vi "FPGA_MAIN.vi"() -> ()   [LabVIEW 2009]
doc: "IRQ Guide:\n3 - SICK IRQ - used to wait at the beginning to set baud rate, and then later to ask for data from the SICK.\n4 - Simple Serial Read IRQ - Used to wait at the beginning to set GPS port baud rate, and then later used to read a data byte from the serial port.\n5 - Simple Serial Clear RX FIFO IRQ - Used to clear the GPS port rx FIFO"
uses:
  <vilib>/LabVIEW Targets/FPGA/cRIO/shared/nicrio_ModuleControls/nicrio_cRIO-9871_BaudRateEnum.ctl
  <vilib>/LabVIEW Targets/FPGA/cRIO/shared/nicrio_ModuleControls/nicrio_cRIO-9871_DataBitsEnum.ctl
  <vilib>/LabVIEW Targets/FPGA/cRIO/shared/nicrio_ModuleControls/nicrio_cRIO-9871_StopBitsEnum.ctl
  <vilib>/LabVIEW Targets/FPGA/cRIO/shared/nicrio_ModuleControls/nicrio_cRIO-9871_ParityEnum.ctl
  <vilib>/LabVIEW Targets/FPGA/cRIO/shared/nicrio_ModuleControls/nicrio_cRIO-9871_FlowControlEnum.ctl
  <vilib>/eio/EIONode/EIONode.xnode
  <vilib>/rvi/eio/nirviEIOImplementation/nirviEIOImplementation.xnode
  <vilib>/rvi/eio/common/nirviEmuTemplateMethod_noerrors.vi
  <vilib>/rvi/eio/common/nirviEmuClasses.ctl
  <vilib>/rvi/Arithmetic/AddSubMult/XNode/nirviSatArithmetic.xnode
  <vilib>/rvi/DataTransferAndStorage/Container/XNode/niFpgaContainer.xnode
  <vilib>/rvi/interface/RandomDataEmulation/niFpgaRandomDataHandleErrors.vi
  <vilib>/rvi/interface/RandomDataEmulation/nirviRandomDataFPGAFIFO.vi
  <vilib>/rvi/DataTransferAndStorage/Container/Common/niFpgaContainerMethod.ctl
  <vilib>/rvi/DataTransferAndStorage/Container/Common/niFpgaTransferTypeControl.ctl
  <vilib>/rvi/Memory/Memory_Emulation/nirvimemoryEmulationManagerCache_GetValue.vi
  <vilib>/rvi/Memory/Memory_Emulation/nirvimemoryEmulationManagerCache_InsertValue.vi
  <vilib>/rvi/DataTransferAndStorage/Container/Common/niFpgaContainerGetUniqueNameForEmu.vi
  <vilib>/Utility/error.llb/Clear Errors.vi
  <vilib>/rvi/Memory/Memory_Emulation/nirvimemoryEmulationManagerCache_SetValue.vi
  <vilib>/eio/EIOPropertyNode/EIOPropertyNode.xnode
  <vilib>/rvi/eio/nirviEIOPropertyImplementation/nirviEIOPropertyImplementation.xnode
  <vilib>/rvi/eio/common/nirviEmuTemplatePropertySet_errors.vi
  <vilib>/eio/EIOMethodNode/EIOMethodNode.xnode
  <vilib>/rvi/eio/nirviEIOMethodImplementation/nirviEIOMethodImplementation.xnode
  <vilib>/rvi/eio/common/nirviEmuTemplateMethod_errors.vi
  SICK VI's/SICK Reader States.ctl
  <vilib>/rvi/eio/common/nirviEmuTemplatePropertyGet_errors.vi
panel:
  in  "Position Reset":bool
  in  "Velocity Interval (uSec)":u32=1000
  out "Right Position (Counts)":i32
  out "Right Acceleration (Counts/Interval)":i32
  out "Right Velocity (Counts/Interval)":i32
  out "Left Position (Counts)":i32
  out "Left Acceleration (Counts/Interval)":i32
  out "Left Velocity (Counts/Interval)":i32
  in  "Safety Light LED ON/OFF/BLINK":u8
  in  "That Was Easy Duration":u32 caption="That Was Easy Duration (ms)"
  in  "Mod2/DIO15:8":u8
  out "Waveform Chart (Turn)":i32(graph)
  out "High Pulse Length (Turn)":i32
  out "Low Pulse Length (Turn)":i32
  out "Pulse Period (Turn)":i32
  out "Waveform Chart (Throttle)":i32(graph)
  out "High Pulse Length (Throttle)":i32
  out "Low Pulse Length (Throttle)":i32
  out "Pulse Period (Throttle)":i32
  out "Debounced BTTN1":bool
  out "Debounced SW2":bool
  out "Debounced SW1":bool
  in  "LED7 ON/OFF/BLINK":u8
  in  "LED6 ON/OFF/BLINK":u8
  in  "LED5 ON/OFF/BLINK":u8
  in  "LED4 ON/OFF/BLINK":u8
  in  "LED3 ON/OFF/BLINK":u8
  in  "LED2 ON/OFF/BLINK":u8
  in  "LED1 ON/OFF/BLINK":u8
  in  "GO LED ON/OFF/BLINK":u8
  in  "Safety LED ON/OFF/BLINK":u8
  in  "Sleep":bool
  out "Chassis Temperature":i16
  out "Output Started":bool
  out "Output Halted":bool
  in  "GPS Read Timeout (us)":i32
  out "Bytes at Port?":bool
  out "Current Buffer":u8[](array[numeric])
  out "GPS Data":u8[](array[numeric])
  out "New GPS Data":bool
  out "GPS error out":errorcluster
  out "Analog Readings":fxp<+/-,16,7>[](array[numeric]) format="%.12g"
  out "Debounced Init Switch":bool
  out "Debounced Go Button":bool
  out "Debounced Safety Switch":bool
  in  "Debounce Timeout":i32=100
  in  "LED Multiple":u32=500
  in  "Init LED ON/OFF/BLINK":u8
  in  "EN mask overflow bytes":bool
  in  "En overflow replacement":bool
  out "Read Period":u32
  out "Tick count":u32
  out "error out 2":errorcluster
  out "Read data error":errorcluster
  in  "Read/Write Timeout (ms)":i32
  in  "Bytes at Port Timeout (us)":i32
  in  "Overflow Reading":u16
  out "No Data (timeout)":bool
  out "Correct Response Read?":bool
  out "Current response length":u8
  out "Timed Out":bool
  out "Initialization error":errorcluster
  in  "Set new baud rate wait (usec)":u32
  out "Baud Rate":T1=enum."38.4 kbps"
  out "RT commands timeout":bool
  out "Pre-initialization error":errorcluster
  out "Commands stored":bool
  out "Pre-initialization success":bool
  out "Initialization success":bool
  out "Compass Period (ms)":u16
  in  "Compass Tick Count(mSec)":u16
  out "Compass Heartbeat":bool
  out "Compass comma count":i32
  out "Compass read count":i32
  in  "Compass Timeout (ms)":i32=150
  out "Compass error out":errorcluster
  out "pitch buffer":u8[](array[numeric])
  out "heading data":u8[](array[numeric])
  out "heading buffer":u8[](array[numeric])
  out "roll data":u8[](array[numeric])
  out "roll buffer":u8[](array[numeric])
  out "pitch data":u8[](array[numeric])
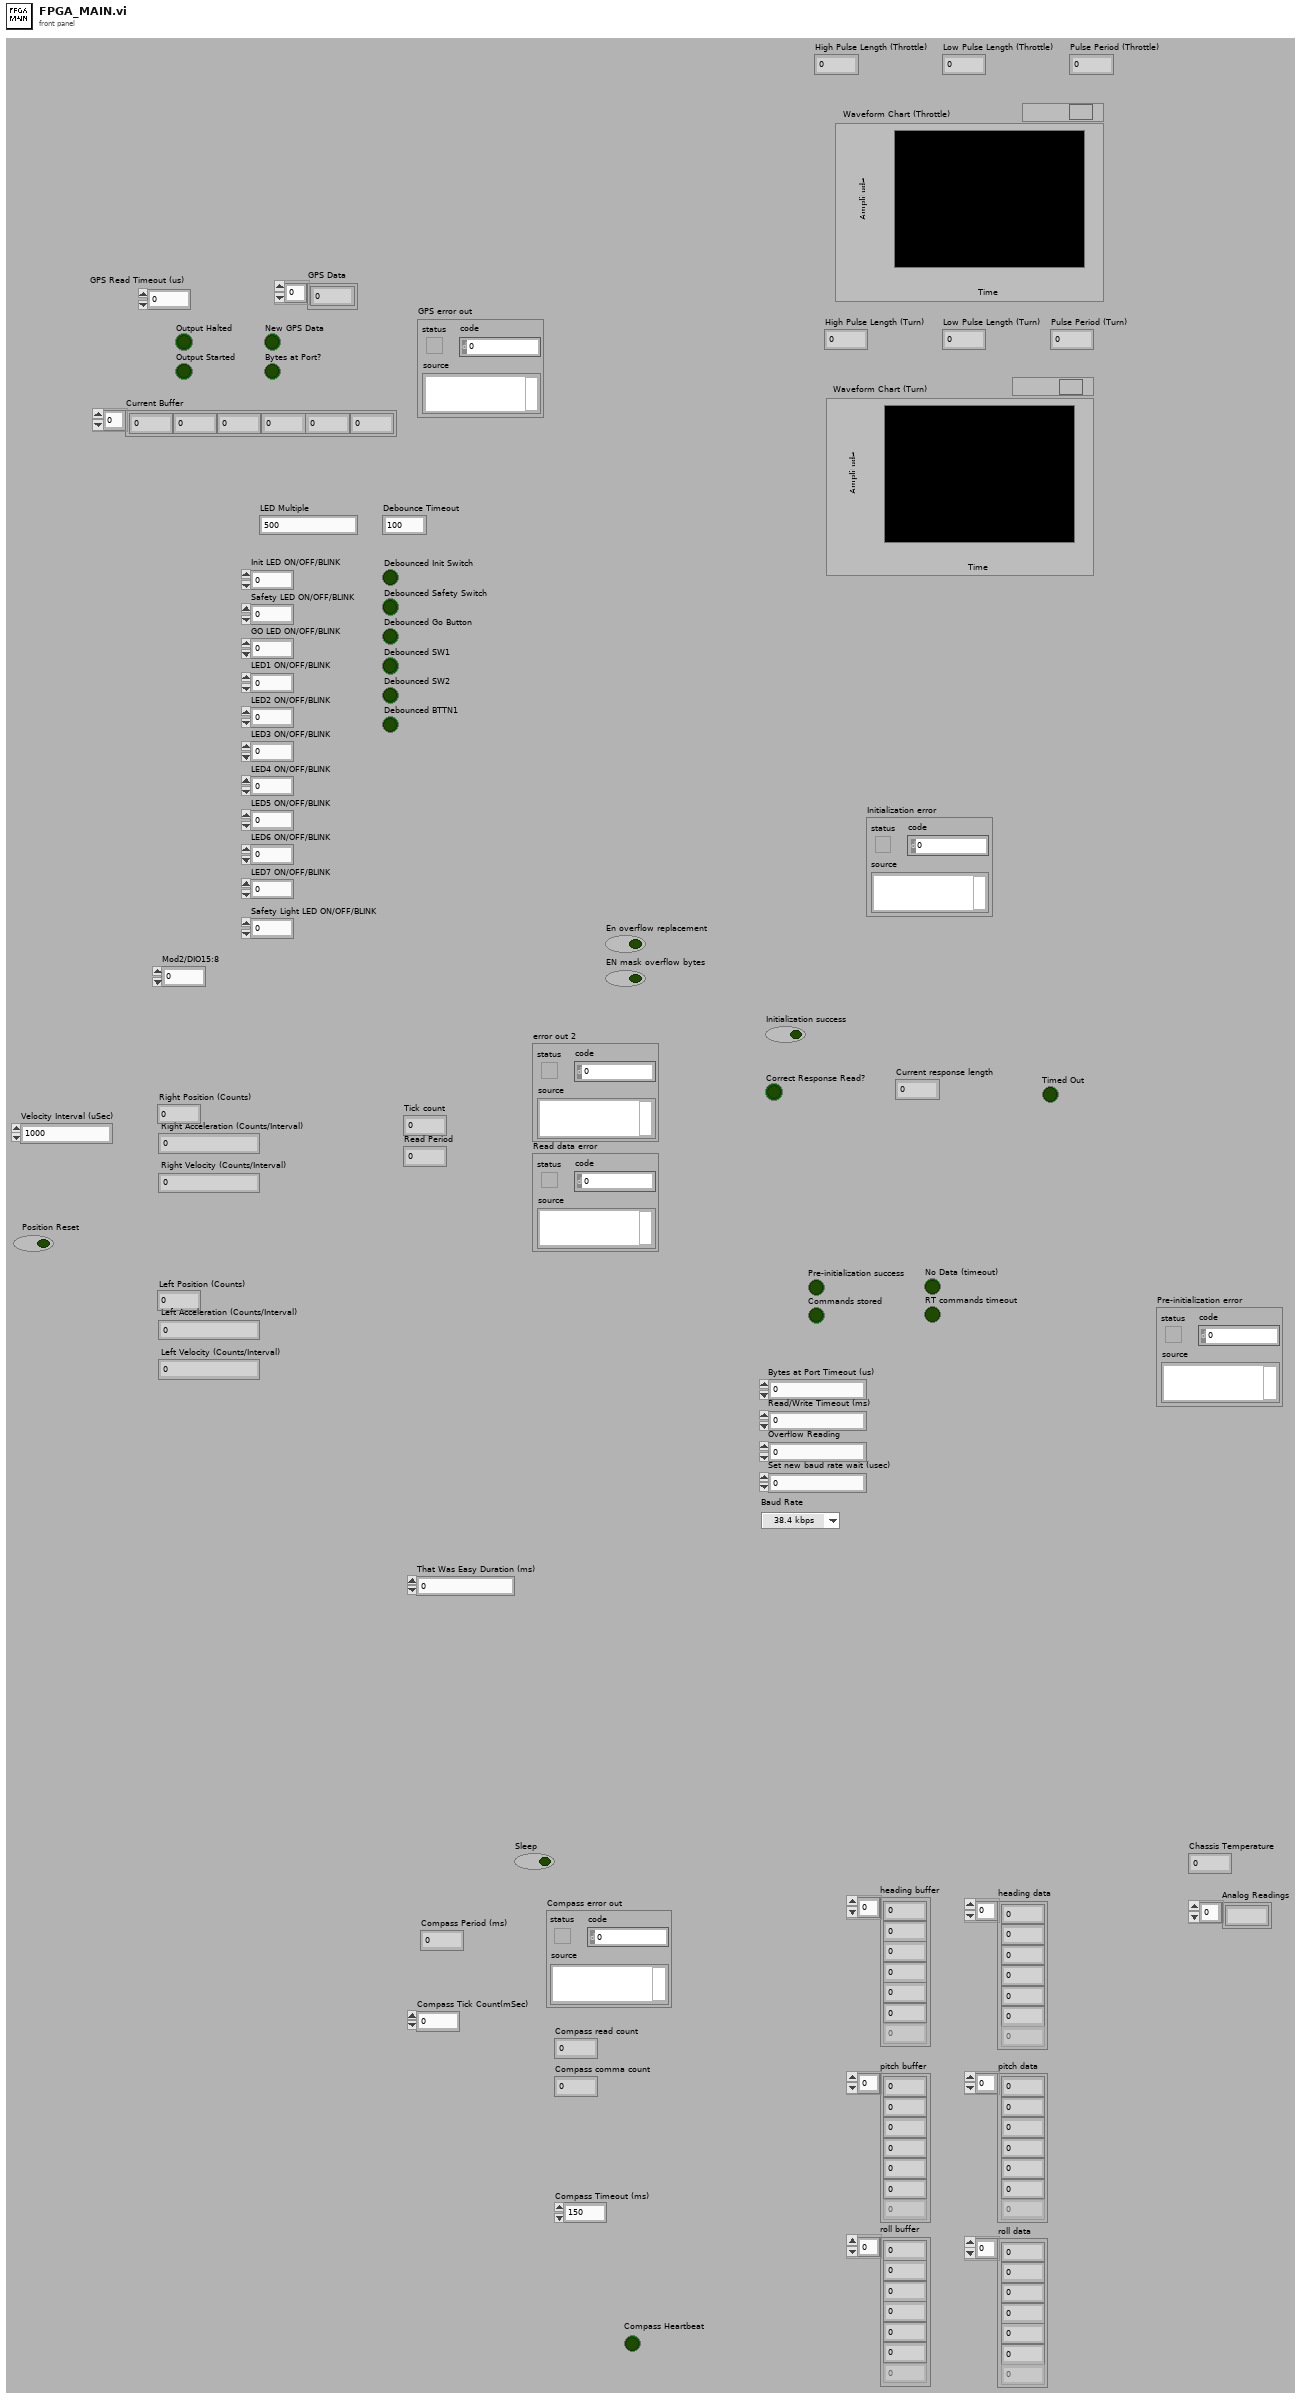
[diagram p1: front panel]
types:
  T1 = typedef "nicrio_cRIO-9871_BaudRateEnum.ctl" = enum16{"75 bps", "110 bps", "134 bps", "150 bps", "300 bps", "600 bps", "1200 bps", "1800 bps", "2400 bps", "4800 bps", "7200 bps", "9600 bps", "14.4 kbps", "19.2 kbps", "28.8 kbps", "38.4 kbps", "57.6 kbps", "115.2 kbps", "230.4 kbps", "460.8 kbps", "921.6 kbps"}
  T2 = typedef "nicrio_cRIO-9871_FlowControlEnum.ctl" = enum8{"None", "Software (XON / XOFF)", "Hardware (RTS / CTS)"}
  T3 = typedef "nicrio_cRIO-9871_ParityEnum.ctl" = enum8{"None", "Odd", "Even", "Mark", "Space"}
  T4 = typedef "nicrio_cRIO-9871_StopBitsEnum.ctl" = enum8{"1", "1.5", "2"}
  T5 = typedef "nicrio_cRIO-9871_DataBitsEnum.ctl" = enum8{"5", "6", "7", "8"}
  T6 = typedef "nirviEmuClasses.ctl" = enum16{"IO Read", "IO Write", "Method", "Property Read", "Property Write"}
  T7 = typedef "niFpgaContainerMethod.ctl" = enum16{"Write", "Read", "Clear", "Get Number of Elements to Write", "Get Number of Elements to Read", "Enable", "Disable", "Flush and Disable", "Get Stream State"}
  T8 = typedef "niFpgaTransferTypeControl.ctl" = enum16{"Target-Scoped", "Host to Target - DMA", "Target to Host - DMA", "Peer to Peer Reader", "Peer to Peer Writer", "Bidirectional"}
  T9 = typedef "SICK Reader States.ctl" = enum16{"Search for 02", "Search for Header", "Read Data"}
  T10 = enum16{"Search for LF", "Read heading", "Read pitch", "Read roll"}
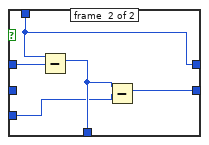
[diagram p2: hidden frame]
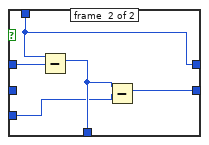
[diagram p3: hidden frame]
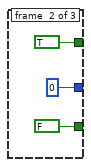
[diagram p4: hidden frame]
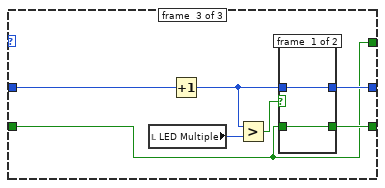
[diagram p5: hidden frame]
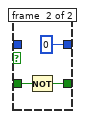
[diagram p6: hidden frame]
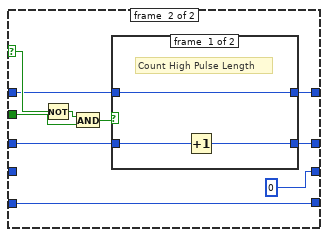
[diagram p8: hidden frame]
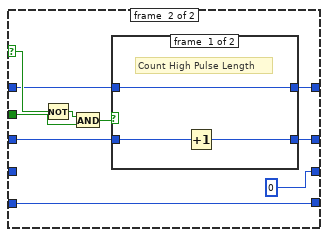
[diagram p11: hidden frame]
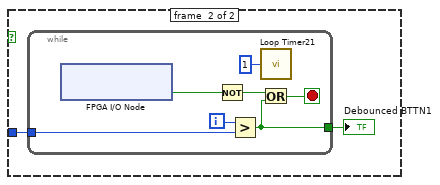
[diagram p13: hidden frame]
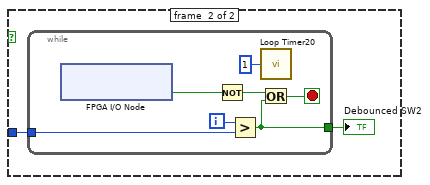
[diagram p14: hidden frame]
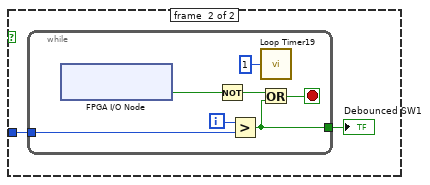
[diagram p15: hidden frame]
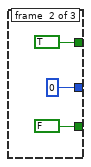
[diagram p16: hidden frame]
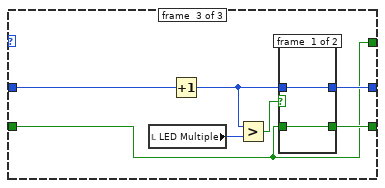
[diagram p17: hidden frame]
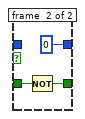
[diagram p18: hidden frame]
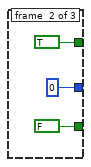
[diagram p19: hidden frame]
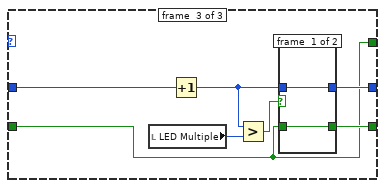
[diagram p20: hidden frame]
diagram:
  # "Debouncing Loops"
  n1 = while "LED3 Loop" {
    shift-right: [w52] -> _
    shift-left: u32 0 -> [w53]
    shift-right: [w51] -> _
    shift-left: FALSE -> [w50]
    stop <- FALSE stop-if-true
    n2 = call "Loop Timer14"("Count(mSec)"=u8 1 ("LED Control Loop Period")) -> ()  [unwired: 1 out]
    n3 = case shown="2" "LED3 ON/OFF/BLINK" {
      tunnel: w53 -> [_ _ w77]
      tunnel: [u32 0 u32 0 w76] -> w52
      tunnel: [FALSE FALSE w73] -> w51
      tunnel: w50 -> [_ _ w72]
      tunnel: [FALSE TRUE w72] -> w49
      frame #0 {
      }
      frame #1 {
      }
      frame #2 {
        n4 = local read "LED Multiple"() -> (w71:u32)
        n5 = Increment(x=w77) -> (x+1=w75:u32)
        n6 = Greater?(x=w75, y=w71) -> (0:w74:bool)
        n7 = case shown="True" w74 {
          tunnel: [w79 u32 0] -> w76
          tunnel: w75 -> [w79 _]
          tunnel: [w78 w81] -> w73
          tunnel: w72 -> [w78 w80]
          frame #0 {
          }
          frame #1 {
            n8 = Not(x=w80) -> (.not. x?=w81:bool)
          }
        }
      }
    }
    n9 = xnode "FPGA I/O Node"("Mod2/DIO24"=w49) -> ()  [unwired: 1 in, 1 out]
  }
  n10 = while "LED4 Loop" {
    shift-right: [w89] -> _
    shift-left: u32 0 -> [w90]
    shift-right: [w88] -> _
    shift-left: FALSE -> [w87]
    stop <- FALSE stop-if-true
    n11 = call "Loop Timer15"("Count(mSec)"=u8 1 ("LED Control Loop Period")) -> ()  [unwired: 1 out]
    n12 = case shown="2" "LED4 ON/OFF/BLINK" {
      tunnel: w90 -> [_ _ w114]
      tunnel: [u32 0 u32 0 w113] -> w89
      tunnel: [FALSE FALSE w110] -> w88
      tunnel: w87 -> [_ _ w109]
      tunnel: [FALSE TRUE w109] -> w86
      frame #0 {
      }
      frame #1 {
      }
      frame #2 {
        n13 = local read "LED Multiple"() -> (w108:u32)
        n14 = Increment(x=w114) -> (x+1=w112:u32)
        n15 = Greater?(x=w112, y=w108) -> (0:w111:bool)
        n16 = case shown="True" w111 {
          tunnel: [w116 u32 0] -> w113
          tunnel: w112 -> [w116 _]
          tunnel: [w115 w118] -> w110
          tunnel: w109 -> [w115 w117]
          frame #0 {
          }
          frame #1 {
            n17 = Not(x=w117) -> (.not. x?=w118:bool)
          }
        }
      }
    }
    n18 = xnode "FPGA I/O Node"("Mod2/DIO25"=w86) -> ()  [unwired: 1 in, 1 out]
  }
  n19 = while "LED5 Loop" {
    shift-right: [w126] -> _
    shift-left: u32 0 -> [w127]
    shift-right: [w125] -> _
    shift-left: FALSE -> [w124]
    stop <- FALSE stop-if-true
    n20 = call "Loop Timer16"("Count(mSec)"=u8 1 ("LED Control Loop Period")) -> ()  [unwired: 1 out]
    n21 = case shown="2" "LED5 ON/OFF/BLINK" {
      tunnel: w127 -> [_ _ w151]
      tunnel: [u32 0 u32 0 w150] -> w126
      tunnel: [FALSE FALSE w147] -> w125
      tunnel: w124 -> [_ _ w146]
      tunnel: [FALSE TRUE w146] -> w123
      frame #0 {
      }
      frame #1 {
      }
      frame #2 {
        n22 = local read "LED Multiple"() -> (w145:u32)
        n23 = Increment(x=w151) -> (x+1=w149:u32)
        n24 = Greater?(x=w149, y=w145) -> (0:w148:bool)
        n25 = case shown="True" w148 {
          tunnel: [w153 u32 0] -> w150
          tunnel: w149 -> [w153 _]
          tunnel: [w152 w155] -> w147
          tunnel: w146 -> [w152 w154]
          frame #0 {
          }
          frame #1 {
            n26 = Not(x=w154) -> (.not. x?=w155:bool)
          }
        }
      }
    }
    n27 = xnode "FPGA I/O Node"("Mod2/DIO26"=w123) -> ()  [unwired: 1 in, 1 out]
  }
  n28 = while "LED6 Loop" {
    shift-right: [w163] -> _
    shift-left: u32 0 -> [w164]
    shift-right: [w162] -> _
    shift-left: FALSE -> [w161]
    stop <- FALSE stop-if-true
    n29 = call "Loop Timer17"("Count(mSec)"=u8 1 ("LED Control Loop Period")) -> ()  [unwired: 1 out]
    n30 = case shown="2" "LED6 ON/OFF/BLINK" {
      tunnel: w164 -> [_ _ w188]
      tunnel: [u32 0 u32 0 w187] -> w163
      tunnel: [FALSE FALSE w184] -> w162
      tunnel: w161 -> [_ _ w183]
      tunnel: [FALSE TRUE w183] -> w160
      frame #0 {
      }
      frame #1 {
      }
      frame #2 {
        n31 = local read "LED Multiple"() -> (w182:u32)
        n32 = Increment(x=w188) -> (x+1=w186:u32)
        n33 = Greater?(x=w186, y=w182) -> (0:w185:bool)
        n34 = case shown="True" w185 {
          tunnel: [w190 u32 0] -> w187
          tunnel: w186 -> [w190 _]
          tunnel: [w189 w192] -> w184
          tunnel: w183 -> [w189 w191]
          frame #0 {
          }
          frame #1 {
            n35 = Not(x=w191) -> (.not. x?=w192:bool)
          }
        }
      }
    }
    n36 = xnode "FPGA I/O Node"("Mod2/DIO29"=w160) -> ()  [unwired: 1 in, 1 out]
  }
  n37 = while "LED7 Loop" {
    shift-right: [w200] -> _
    shift-left: u32 0 -> [w201]
    shift-right: [w199] -> _
    shift-left: FALSE -> [w198]
    stop <- FALSE stop-if-true
    n38 = call "Loop Timer18"("Count(mSec)"=u8 1 ("LED Control Loop Period")) -> ()  [unwired: 1 out]
    n39 = case shown="2" "LED7 ON/OFF/BLINK" {
      tunnel: w201 -> [_ _ w225]
      tunnel: [u32 0 u32 0 w224] -> w200
      tunnel: [FALSE FALSE w221] -> w199
      tunnel: w198 -> [_ _ w220]
      tunnel: [FALSE TRUE w220] -> w197
      frame #0 {
      }
      frame #1 {
      }
      frame #2 {
        n40 = local read "LED Multiple"() -> (w219:u32)
        n41 = Increment(x=w225) -> (x+1=w223:u32)
        n42 = Greater?(x=w223, y=w219) -> (0:w222:bool)
        n43 = case shown="True" w222 {
          tunnel: [w227 u32 0] -> w224
          tunnel: w223 -> [w227 _]
          tunnel: [w226 w229] -> w221
          tunnel: w220 -> [w226 w228]
          frame #0 {
          }
          frame #1 {
            n44 = Not(x=w228) -> (.not. x?=w229:bool)
          }
        }
      }
    }
    n45 = xnode "FPGA I/O Node"("Mod2/DIO30"=w197) -> ()  [unwired: 1 in, 1 out]
  }
  n46 = while {
    stop <- FALSE stop-if-true
    n47 = xnode "FPGA I/O Node"() -> ("Mod1/AI0"=w245:fxp<+/-,16,7>)  [unwired: 1 in, 1 out]
    n48 = xnode "FPGA I/O Node"() -> ("Mod1/AI1"=w244:fxp<+/-,16,7>)  [unwired: 1 in, 1 out]
    n49 = xnode "FPGA I/O Node"() -> ("Mod1/AI2"=w243:fxp<+/-,16,7>)  [unwired: 1 in, 1 out]
    n50 = xnode "FPGA I/O Node"() -> ("Mod1/AI3"=w242:fxp<+/-,16,7>)  [unwired: 1 in, 1 out]
    n51 = xnode "FPGA I/O Node"() -> ("Mod1/AI4"=w241:fxp<+/-,16,7>)  [unwired: 1 in, 1 out]
    n52 = xnode "FPGA I/O Node"() -> ("Mod1/AI5"=w240:fxp<+/-,16,7>)  [unwired: 1 in, 1 out]
    n53 = xnode "FPGA I/O Node"() -> ("Mod1/AI6"=w239:fxp<+/-,16,7>)  [unwired: 1 in, 1 out]
    n54 = xnode "FPGA I/O Node"() -> ("Mod1/AI7"=w238:fxp<+/-,16,7>)  [unwired: 1 in, 1 out]
    n55 = xnode "FPGA I/O Node"() -> ("Chassis Temperature"=→"Chassis Temperature":i16)  [unwired: 1 in, 1 out]
    n56 = xnode "FPGA I/O Node"("Sleep"="Sleep") -> ()  [unwired: 1 in, 1 out]
    n57 = Build Array(w245, w244, w243, w242, w241, w240, w239, w238) -> (→"Analog Readings":fxp<+/-,16,7>[])
    n58 = Number To Boolean Array(number="Mod2/DIO15:8") -> (Boolean array=w235:bool[])
    n59 = Index Array(array=w235, index #1=1 ("index")) -> (element #1=w232:bool, element #2=w231:bool)  [unwired: 1 in]
    n60 = xnode "FPGA I/O Node"("Mod2/DIO13"=w232, "Mod2/DIO14"=w231) -> ()  [unwired: 2 in, 2 out]
  }
  n61 = while "LED2 Loop" {
    shift-right: [w466] -> _
    shift-left: u32 0 -> [w467]
    shift-right: [w465] -> _
    shift-left: FALSE -> [w464]
    stop <- FALSE stop-if-true
    n62 = call "Loop Timer13"("Count(mSec)"=u8 1 ("LED Control Loop Period")) -> ()  [unwired: 1 out]
    n63 = case shown="2" "LED2 ON/OFF/BLINK" {
      tunnel: w467 -> [_ _ w491]
      tunnel: [u32 0 u32 0 w490] -> w466
      tunnel: [FALSE FALSE w487] -> w465
      tunnel: w464 -> [_ _ w486]
      tunnel: [FALSE TRUE w486] -> w463
      frame #0 {
      }
      frame #1 {
      }
      frame #2 {
        n64 = local read "LED Multiple"() -> (w485:u32)
        n65 = Increment(x=w491) -> (x+1=w489:u32)
        n66 = Greater?(x=w489, y=w485) -> (0:w488:bool)
        n67 = case shown="True" w488 {
          tunnel: [w493 u32 0] -> w490
          tunnel: w489 -> [w493 _]
          tunnel: [w492 w495] -> w487
          tunnel: w486 -> [w492 w494]
          frame #0 {
          }
          frame #1 {
            n68 = Not(x=w494) -> (.not. x?=w495:bool)
          }
        }
      }
    }
    n69 = xnode "FPGA I/O Node"("Mod2/DIO23"=w463) -> ()  [unwired: 1 in, 1 out]
  }
  n70 = while "Safety Light LED Loop" {
    shift-right: [w503] -> _
    shift-left: u32 0 -> [w504]
    shift-right: [w502] -> _
    shift-left: FALSE -> [w501]
    stop <- FALSE stop-if-true
    n71 = call "Loop Timer24"("Count(mSec)"=u8 1 ("LED Control Loop Period")) -> ()  [unwired: 1 out]
    n72 = case shown="0" "Safety Light LED ON/OFF/BLINK" {
      tunnel: w504 -> [_ _ w528]
      tunnel: [u32 0 u32 0 w527] -> w503
      tunnel: [FALSE FALSE w524] -> w502
      tunnel: w501 -> [_ _ w523]
      tunnel: [FALSE TRUE w523] -> w500
      frame #0 {
      }
      frame #1 {
      }
      frame #2 {
        n73 = local read "LED Multiple"() -> (w522:u32)
        n74 = Increment(x=w528) -> (x+1=w526:u32)
        n75 = Greater?(x=w526, y=w522) -> (0:w525:bool)
        n76 = case shown="True" w525 {
          tunnel: [w530 u32 0] -> w527
          tunnel: w526 -> [w530 _]
          tunnel: [w529 w532] -> w524
          tunnel: w523 -> [w529 w531]
          frame #0 {
          }
          frame #1 {
            n77 = Not(x=w531) -> (.not. x?=w532:bool)
          }
        }
      }
    }
    n78 = xnode "FPGA I/O Node"("Mod2/DIO15"=w500) -> ()  [unwired: 1 in, 1 out]
  }
  n79 = while "GO LED Loop" {
    shift-right: [w540] -> _
    shift-left: u32 0 -> [w541]
    shift-right: [w539] -> _
    shift-left: FALSE -> [w538]
    stop <- FALSE stop-if-true
    # "GO LED"
    n80 = call "Loop Timer11"("Count(mSec)"=u8 1 ("LED Control Loop Period")) -> ()  [unwired: 1 out]
    n81 = case shown="0, Default" "GO LED ON/OFF/BLINK" {
      tunnel: w541 -> [_ _ w565]
      tunnel: [u32 0 u32 0 w564] -> w540
      tunnel: [FALSE FALSE w561] -> w539
      tunnel: w538 -> [_ _ w560]
      tunnel: [FALSE TRUE w560] -> w537
      frame #0 {
      }
      frame #1 {
      }
      frame #2 {
        n82 = local read "LED Multiple"() -> (w559:u32)
        n83 = Increment(x=w565) -> (x+1=w563:u32)
        n84 = Greater?(x=w563, y=w559) -> (0:w562:bool)
        n85 = case shown="True" w562 {
          tunnel: [w567 u32 0] -> w564
          tunnel: w563 -> [w567 _]
          tunnel: [w566 w569] -> w561
          tunnel: w560 -> [w566 w568]
          frame #0 {
          }
          frame #1 {
            n86 = Not(x=w568) -> (.not. x?=w569:bool)
          }
        }
      }
    }
    n87 = xnode "FPGA I/O Node"("Mod2/DIO18"=w537) -> ()  [unwired: 1 in, 1 out]
  }
  n88 = while "LED1 Loop" {
    shift-right: [w577] -> _
    shift-left: u32 0 -> [w578]
    shift-right: [w576] -> _
    shift-left: FALSE -> [w575]
    stop <- FALSE stop-if-true
    n89 = call "Loop Timer12"("Count(mSec)"=u8 1 ("LED Control Loop Period")) -> ()  [unwired: 1 out]
    n90 = case shown="2" "LED1 ON/OFF/BLINK" {
      tunnel: w578 -> [_ _ w602]
      tunnel: [u32 0 u32 0 w601] -> w577
      tunnel: [FALSE FALSE w598] -> w576
      tunnel: w575 -> [_ _ w597]
      tunnel: [FALSE TRUE w597] -> w574
      frame #0 {
      }
      frame #1 {
      }
      frame #2 {
        n91 = local read "LED Multiple"() -> (w596:u32)
        n92 = Increment(x=w602) -> (x+1=w600:u32)
        n93 = Greater?(x=w600, y=w596) -> (0:w599:bool)
        n94 = case shown="True" w599 {
          tunnel: [w604 u32 0] -> w601
          tunnel: w600 -> [w604 _]
          tunnel: [w603 w606] -> w598
          tunnel: w597 -> [w603 w605]
          frame #0 {
          }
          frame #1 {
            n95 = Not(x=w605) -> (.not. x?=w606:bool)
          }
        }
      }
    }
    n96 = xnode "FPGA I/O Node"("Mod2/DIO22"=w574) -> ()  [unwired: 1 in, 1 out]
  }
  n97 = while "Safety LED Loop" {
    shift-right: [w614] -> _
    shift-left: u32 0 -> [w615]
    shift-right: [w613] -> _
    shift-left: FALSE -> [w612]
    stop <- FALSE stop-if-true
    # "Safety LED"
    n98 = call "Loop Timer10"("Count(mSec)"=u8 1 ("LED Control Loop Period")) -> ()  [unwired: 1 out]
    n99 = case shown="2" "Safety LED ON/OFF/BLINK" {
      tunnel: w615 -> [_ _ w639]
      tunnel: [u32 0 u32 0 w638] -> w614
      tunnel: [FALSE FALSE w635] -> w613
      tunnel: w612 -> [_ _ w634]
      tunnel: [FALSE TRUE w634] -> w611
      frame #0 {
      }
      frame #1 {
      }
      frame #2 {
        n100 = local read "LED Multiple"() -> (w633:u32)
        n101 = Increment(x=w639) -> (x+1=w637:u32)
        n102 = Greater?(x=w637, y=w633) -> (0:w636:bool)
        n103 = case shown="True" w636 {
          tunnel: [w641 u32 0] -> w638
          tunnel: w637 -> [w641 _]
          tunnel: [w640 w643] -> w635
          tunnel: w634 -> [w640 w642]
          frame #0 {
          }
          frame #1 {
            n104 = Not(x=w642) -> (.not. x?=w643:bool)
          }
        }
      }
    }
    n105 = xnode "FPGA I/O Node"("Mod2/DIO17"=w611) -> ()  [unwired: 1 in, 1 out]
  }
  n106 = while "Init LED Loop" {
    shift-right: [w651] -> _
    shift-left: u32 0 -> [w652]
    shift-right: [w650] -> _
    shift-left: FALSE -> [w649]
    stop <- FALSE stop-if-true
    # "Init LED"
    n107 = call "Loop Timer4"("Count(mSec)"=u8 1 ("LED Control Loop Period")) -> ()  [unwired: 1 out]
    n108 = case shown="2" "Init LED ON/OFF/BLINK" {
      tunnel: w652 -> [_ _ w676]
      tunnel: [u32 0 u32 0 w675] -> w651
      tunnel: [FALSE FALSE w672] -> w650
      tunnel: w649 -> [_ _ w671]
      tunnel: [FALSE TRUE w671] -> w648
      frame #0 {
      }
      frame #1 {
      }
      frame #2 {
        n109 = local read "LED Multiple"() -> (w670:u32)
        n110 = Increment(x=w676) -> (x+1=w674:u32)
        n111 = Greater?(x=w674, y=w670) -> (0:w673:bool)
        n112 = case shown="True" w673 {
          tunnel: [w678 u32 0] -> w675
          tunnel: w674 -> [w678 _]
          tunnel: [w677 w680] -> w672
          tunnel: w671 -> [w677 w679]
          frame #0 {
          }
          frame #1 {
            n113 = Not(x=w679) -> (.not. x?=w680:bool)
          }
        }
      }
    }
    n114 = xnode "FPGA I/O Node"("Mod2/DIO16"=w648) -> ()  [unwired: 1 in, 1 out]
  }
  n115 = while {
    stop <- FALSE stop-if-true
    n116 = flat-sequence {
      tunnel: [w688] -> w685
      tunnel: w685 -> [w928]
      tunnel: [w927] -> w683
      tunnel: w683 -> [w945]
      tunnel: [w945] -> w682
      tunnel: w682 -> [w1198]
      frame #0 {
        w686 = FALSE ("Initialization complete")
        n117 = local write "RT commands timeout"(w686) -> ()
        n118 = local write "Pre-initialization success"(w686) -> ()
        n119 = local write "Commands stored"(w686) -> ()
        n120 = local write "No Data (timeout)"(w686) -> ()
        "Initialization success" <- w686
      }
      frame #1 {
        n121 = flat-sequence {
          tunnel: [w863] -> w687
          tunnel: [TRUE] -> w689
          frame #0 {
            w865 = nicrio_cRIO-9871_BaudRateEnum."38.4 kbps" ("Baud Rate")
            # "Set baud rate to 38.4 kbps and tell it to cease continuous data output to prevent the FPGA from mixing up data messages and command responses"
            n122 = call "Wait"("Count(uSec)"="Set new baud rate wait (usec)") -> ()  [unwired: 1 out]
            n123 = xnode "FPGA I/O Property Node"("Baud Rate"=w865, "Data Bits"=nicrio_cRIO-9871_DataBitsEnum."8", "Stop Bits"=nicrio_cRIO-9871_StopBitsEnum."1", "Parity"=nicrio_cRIO-9871_ParityEnum."None", "Flow Control"=nicrio_cRIO-9871_FlowControlEnum."None") -> ("error out"=w862:errorcluster)  [unwired: 2 in, 1 out]
            n124 = xnode "FPGA I/O Method Node"("error in"=w862) -> ("error out"=w863:errorcluster)  [unwired: 1 in, 1 out]
            "Baud Rate" <- w865
          }
        }
        n125 = flat-sequence {
          tunnel: errorcluster {"status"=FALSE, "code"=0, "source"=""} ("error out") -> [w694]
          tunnel: [w694] -> w693
          tunnel: w693 -> [w699]
          tunnel: [w698] -> w691
          tunnel: [TRUE] -> w690
          frame #0 {
            n126 = call "Interrupt"("Wait Until Cleared"=TRUE, "IRQ Number"=u8 3) -> ()  [unwired: 1 out]
          }
          frame #1 {
            n127 = for "Read all the commands from the RT to memory" {
              N: 160 -> [_]
              tunnel: w699 -> [w706]
              tunnel: [w705] -> w698
              i -> [w702]
              n128 = local read "Read/Write Timeout (ms)"() -> (w704:i32)
              n129 = xnode ("FIFO Read")("Timeout"=w704, "error in (no error)"=w706) -> ("Element"=w708:u8, "Timed Out?"=→"RT commands timeout":bool, "error out"=w707:errorcluster)  [unwired: 1 in, 1 out]
              n130 = To Unsigned Long Integer(number=w702) -> (unsigned 32bit integer=w701:u32)
              n131 = xnode ("Memory Write")("Address"=w701, "Data"=w708, "error in (no error)"=w707) -> ("error out"=w705:errorcluster)  [unwired: 1 in, 1 out]
            }
          }
        }
        n132 = Select(t=w687, s=w687, f=w691) -> (s? t:f=w688:errorcluster)
        "Pre-initialization error" <- w688
        "Commands stored" <- w690
        "Pre-initialization success" <- w689
      }
      frame #2 {
        n133 = case shown="No Error" w928 {
          selector: w928 -> [w929 w944]
          tunnel: [w930 w944] -> w927
          frame #0 {
            n134 = for {
              N: 5 -> [_]
              shift-right: [w934] -> w930
              shift-left: w929 -> [w935]
              i -> [w933]
              n135 = To Unsigned Long Integer(number=w933) -> (unsigned 32bit integer=w932:u32)
              n136 = while {
                tunnel: w935 -> [w939]
                tunnel: [w941] -> w934
                tunnel: w932 -> [w936]
                stop <- w942 stop-if-true
                n137 = local read "Read/Write Timeout (ms)"() -> (w937:i32)
                n138 = call "FPGA_SICK Write Command.vi"("error in (no error)"=w939, "Read/Write Timeout (ms)"=w937, "Command index"=w936) -> ("error out"=w938:errorcluster)  [unwired: 8 out]
                n139 = call "FPGA_SICK Read Response.vi"("error in (no error)"=w938, "Timeout (ms)"=w937, "Response Index"=w936) -> ("error out"=w941:errorcluster, "Timed Out"=→"Timed Out":bool, "Current response length"=→"Current response length":u8, "Correct Response Read?"=w942:bool)  [unwired: 5 out]
                "Correct Response Read?" <- w942
              }
            }
          }
          frame #1 {
          }
        }
        "Initialization error" <- w927
      }
      frame #3 {
        n140 = local write "Initialization success"(TRUE ("Initialization complete")) -> ()
        n141 = call "Wait2"("Count(mSec)"=u8 100 ("Count(Ticks)")) -> ()  [unwired: 1 out]
        n142 = for {
          N: 181 -> [_]
          tunnel: u16 0 ("Data") -> [w1073]
          i -> [w1075]
          n143 = To Unsigned Long Integer(number=w1075) -> (unsigned 32bit integer=w1074:u32)
          n144 = xnode ("Memory Write")("Address"=w1074, "Data"=w1073) -> ()  [unwired: 1 in, 1 out]
        }
        n145 = xnode ("Memory Write")("Address"=u32 0, "Data"="Overflow Reading") -> ()  [unwired: 1 in, 1 out]
      }
      frame #4 {
        n146 = case shown="No Error" w1198 {
          selector: w1198 -> [_ w1837]
          tunnel: [w1199 w1837] -> w1197
          frame #0 {
            n147 = while {
              tunnel: errorcluster {"status"=FALSE, "code"=0, "source"=""} ("error out") -> [w1206]
              stop <- FALSE stop-if-true
              n148 = flat-sequence {
                tunnel: w1206 -> [w1208]
                tunnel: [w1208] -> w1207
                tunnel: w1207 -> [w1212]
                tunnel: [w1211] -> w1205
                frame #0 {
                  n149 = call "Interrupt2"("Wait Until Cleared"=TRUE, "IRQ Number"=u8 3) -> ()  [unwired: 1 out]
                }
                frame #1 {
                  n150 = for {
                    N: 181 -> [_]
                    tunnel: w1212 -> [w1218]
                    tunnel: [w1214] -> w1211
                    i -> [w1220]
                    n151 = To Unsigned Long Integer(number=w1220) -> (unsigned 32bit integer=w1219:u32)
                    n152 = xnode ("Memory Read")("Address"=w1219, "error in (no error)"=w1218) -> ("Data"=w1217:u16, "error out"=w1215:errorcluster)  [unwired: 1 in, 1 out]
                    n153 = local read "Read/Write Timeout (ms)"() -> (w1216:i32)
                    n154 = xnode ("FIFO Write")("Element"=w1217, "Timeout"=w1216, "error in (no error)"=w1215) -> ("error out"=w1214:errorcluster)  [unwired: 1 in, 2 out]
                  }
                }
              }
              "error out 2" <- w1205
            }
            n155 = while {
              tunnel: u8[] [128, 110, 1, 176, 181, 0] -> [w1378]
              tunnel: errorcluster {"status"=FALSE, "code"=0, "source"=""} ("error out") -> [w1377]
              shift-right: [w1376] -> _
              shift-left: SICK_Reader_States."Search for 02" ("SICK Reader States") -> [w1379]
              tunnel: [w1375] -> w1199
              stop <- FALSE stop-if-true
              n156 = case shown="\"Read Data\"" w1379 {
                tunnel: w1378 -> [_ w1459 _]
                tunnel: w1377 -> [w1389 w1458 w1546]
                tunnel: [w1387 w1457 w1543] -> w1375
                tunnel: [w1380 w1455 SICK_Reader_States."Search for 02" ("SICK Reader States")] -> w1376
                frame #0 {
                  n157 = while {
                    tunnel: [w1393] -> w1388
                    tunnel: w1389 -> [w1391]
                    i -> [w1395]
                    stop <- w1397 stop-if-true
                    n158 = xnode "FPGA I/O Property Node"("error in"=w1391) -> ("error out"=w1393:errorcluster, "Bytes at Port"=w1398:u8)  [unwired: 1 in, 1 out]
                    n159 = Not Equal To 0?(x=w1398) -> (x != 0?=w1396:bool)
                    n160 = local read "Bytes at Port Timeout (us)"() -> (w1392:i32)
                    n161 = Greater Or Equal?(x=w1395, y=w1392) -> (x >= y?=w1390:bool)
                    n162 = local write "No Data (timeout)"(w1390) -> ()
                    n163 = Or(x=w1396, y=w1390) -> (x .or. y?=w1397:bool)
                    n164 = call "Loop Timer"("Count(uSec)"=u8 1) -> ()  [unwired: 1 out]
                  }
                  n165 = local read "Read/Write Timeout (ms)"() -> (w1386:i32)
                  n166 = xnode "FPGA I/O Method Node"("error in"=w1388, "Timeout (ms)"=w1386) -> ("error out"=w1387:errorcluster, "Data"=w1385:u8)  [unwired: 1 in, 2 out]
                  n167 = Equal?(x=w1385, y=u8 2) -> (x = y?=w1383:bool)
                  n168 = Select(t=SICK_Reader_States."Search for Header" ("SICK Reader States"), s=w1383, f=SICK_Reader_States."Search for 02" ("SICK Reader States")) -> (s? t:f=w1380:T9)
                }
                frame #1 {
                  n169 = while {
                    tunnel: w1459 -> [w1471] mode=indexing
                    tunnel: w1458 -> [w1473]
                    tunnel: [w1472] -> w1457
                    shift-right: [w1467] -> _
                    shift-left: TRUE ("x = y?") -> [w1469]
                    tunnel: [w1462] -> w1455
                    i -> [w1466]
                    stop <- w1464 continue-if-true
                    n170 = while {
                      tunnel: [w1479] -> w1474
                      tunnel: w1473 -> [w1478]
                      i -> [w1481]
                      stop <- w1483 stop-if-true
                      n171 = xnode "FPGA I/O Property Node"("error in"=w1478) -> ("error out"=w1479:errorcluster, "Bytes at Port"=w1484:u8)  [unwired: 1 in, 1 out]
                      n172 = local read "Bytes at Port Timeout (us)"() -> (w1477:i32)
                      n173 = Not Equal To 0?(x=w1484) -> (x != 0?=w1482:bool)
                      n174 = Greater Or Equal?(x=w1481, y=w1477) -> (x >= y?=w1476:bool)
                      n175 = local write "No Data (timeout)"(w1476) -> ()
                      n176 = Or(x=w1482, y=w1476) -> (x .or. y?=w1483:bool)
                      n177 = call "Loop Timer2"("Count(uSec)"=u8 1) -> ()  [unwired: 1 out]
                    }
                    n178 = local read "Read/Write Timeout (ms)"() -> (w1470:i32)
                    n179 = xnode "FPGA I/O Method Node"("error in"=w1474, "Timeout (ms)"=w1470) -> ("error out"=w1472:errorcluster, "Data"=w1475:u8)  [unwired: 1 in, 2 out]
                    n180 = Equal?(x=w1475, y=w1471) -> (x = y?=w1468:bool)
                    n181 = And(x=w1469, y=w1468) -> (x .and. y?=w1467:bool)
                    n182 = Less?(x=w1466, y=5) -> (x < y?=w1463:bool)
                    n183 = And(x=w1463, y=w1467) -> (x .and. y?=w1464:bool)
                    n184 = Select(t=SICK_Reader_States."Search for 02" ("SICK Reader States"), s=w1463, f=SICK_Reader_States."Read Data" ("SICK Reader States")) -> (s? t:f=w1462:T9)
                  }
                }
                frame #2 {
                  n185 = flat-sequence {
                    tunnel: [w1547] -> w1541
                    tunnel: w1541 -> [w1550]
                    frame #0 {
                      n186 = local read "Tick count"() -> (w1547:u32)
                    }
                    frame #1 {
                      n187 = call "Tick Count2"() -> ("Tick Count(uSec)"=w1548:u32)
                      "Tick count" <- w1548
                      n188 = Subtract(x=w1548, y=w1550) -> (x-y=→"Read Period":u32)
                    }
                  }
                  n189 = while {
                    tunnel: w1546 -> [w1568]
                    tunnel: [w1554] -> w1542
                    i -> [w1557]
                    stop <- w1561 stop-if-true
                    n190 = while {
                      tunnel: [w1735] -> w1569
                      tunnel: w1568 -> [w1734]
                      tunnel: [w1731] -> w1558
                      i -> [w1737]
                      stop <- w1739 stop-if-true
                      n191 = xnode "FPGA I/O Property Node"("error in"=w1734) -> ("error out"=w1735:errorcluster, "Bytes at Port"=w1740:u8)  [unwired: 1 in, 1 out]
                      n192 = Greater Or Equal?(x=w1740, y=u8 2 ("x")) -> (x >= y?=w1738:bool)
                      n193 = local read "Bytes at Port Timeout (us)"() -> (w1733:i32)
                      n194 = Greater Or Equal?(x=w1737, y=w1733) -> (x >= y?=w1731:bool)
                      n195 = local write "No Data (timeout)"(w1731) -> ()
                      n196 = Compound Arithmetic op=OR(w1738, w1731) -> (w1739:bool)
                      n197 = call "Loop Timer3"("Count(uSec)"=u8 1) -> ()  [unwired: 1 out]
                    }
                    n198 = local read "Read/Write Timeout (ms)"() -> (w1559:i32)
                    n199 = xnode "FPGA I/O Method Node"("error in"=w1569, "Timeout (ms)"=w1559) -> ("error out"=w1567:errorcluster, "Data"=w1565:u8)  [unwired: 1 in, 2 out]
                    n200 = xnode "FPGA I/O Method Node"("error in"=w1567, "Timeout (ms)"=w1559) -> ("error out"=w1555:errorcluster, "Data"=w1566:u8)  [unwired: 1 in, 2 out]
                    n201 = local read "No Data (timeout)"() -> (w1560:bool)
                    n202 = Join Numbers(hi=w1566, lo=w1565) -> ((hi.lo)=w1564:u16)
                    n203 = Greater Or Equal?(x=w1557, y=180) -> (x >= y?=w1562:bool)
                    n204 = To Unsigned Long Integer(number=w1557) -> (unsigned 32bit integer=w1556:u32)
                    n205 = call "FPGA_SICK Check for overflows.vi"("EN mask overflow bytes"="EN mask overflow bytes", "Data chunk in"=w1564, "En overflow replacement"="En overflow replacement") -> ("Data chunk out"=w1551:u16)
                    n206 = Compound Arithmetic op=OR(w1558, w1560, w1562) -> (w1561:bool)
                    n207 = xnode ("Memory Write")("Address"=w1556, "Data"=w1551, "error in (no error)"=w1555) -> ("error out"=w1554:errorcluster)  [unwired: 1 in, 1 out]
                  }
                  n208 = for {
                    N: 3 -> [_]
                    tunnel: w1542 -> [w1799]
                    tunnel: [w1798] -> w1543
                    n209 = local read "Read/Write Timeout (ms)"() -> (w1797:i32)
                    n210 = xnode "FPGA I/O Method Node"("error in"=w1799, "Timeout (ms)"=w1797) -> ("error out"=w1798:errorcluster)  [unwired: 1 in, 3 out]
                  }
                }
              }
            }
          }
          frame #1 {
          }
        }
        "Read data error" <- w1197
      }
    }
  }
  n211 = while {
    stop <- FALSE stop-if-true
    n212 = flat-sequence "Compass" {
      tunnel: [w1846] -> w1839
      tunnel: w1839 -> [w1913]
      frame #0 {
        n213 = Initialize Array(u8 32 ("y"), 6 ("dimension size")) -> (→"roll buffer":u8[])
        n214 = Initialize Array(u8 32 ("y"), 6 ("dimension size")) -> (→"pitch data":u8[])
        n215 = Initialize Array(u8 32 ("y"), 6 ("dimension size")) -> (→"heading buffer":u8[])
        n216 = Initialize Array(u8 32 ("y"), 6 ("dimension size")) -> (→"roll data":u8[])
        n217 = Initialize Array(u8 32 ("y"), 6 ("dimension size")) -> (→"heading data":u8[])
        n218 = Initialize Array(u8 32 ("y"), 6 ("dimension size")) -> (→"pitch buffer":u8[])
        n219 = xnode "FPGA I/O Property Node"("Baud Rate"=nicrio_cRIO-9871_BaudRateEnum."19.2 kbps", "Data Bits"=nicrio_cRIO-9871_DataBitsEnum."8", "Stop Bits"=nicrio_cRIO-9871_StopBitsEnum."1", "Parity"=nicrio_cRIO-9871_ParityEnum."None", "Flow Control"=nicrio_cRIO-9871_FlowControlEnum."None") -> ("error out"=w1846:errorcluster)  [unwired: 2 in, 1 out]
        "Compass Heartbeat" <- FALSE ("SICK Heartbeat")
      }
      frame #1 {
        n220 = while {
          shift-right: [w1918] -> _
          shift-left: T10."Search for LF" ("Main states") -> [w1919]
          tunnel: [w1915] -> w1912
          tunnel: w1913 -> [w1914]
          stop <- w1915 stop-if-true
          n221 = while {
            tunnel: [w1962] -> w1922
            tunnel: w1914 -> [w1960]
            stop <- w1963 continue-if-true
            n222 = xnode "FPGA I/O Property Node"("error in"=w1960) -> ("error out"=w1962:errorcluster, "Bytes at Port"=w1961:u8)  [unwired: 1 in, 1 out]
            n223 = Equal To 0?(x=w1961) -> (x = 0?=w1963:bool)
          }
          n224 = xnode "FPGA I/O Method Node"("error in"=w1922, "Timeout (ms)"="Compass Timeout (ms)") -> ("error out"=w1916:errorcluster, "Data"=w1920:u8)  [unwired: 1 in, 2 out]
          n225 = Select(t=errorcluster {"status"=TRUE, "code"=1, "source"="Q error: Compass read byte failed. \nCheck wiring or reinitialize"} ("error out"), s=w1916, f=w1916) -> (s? t:f=w1915:errorcluster)
          n226 = case shown="\"Read heading\"" w1919 {
            tunnel: w1920 -> [w1998 w2002 w2040 w2073]
            tunnel: [w1995 w2003 w2041 w2074] -> w1918
            frame #0 {
              w1988 = 0
              n227 = local write "Compass comma count"(w1988) -> ()
              n228 = local write "Compass read count"(w1988) -> ()
              n229 = Initialize Array(u8 32 ("y"), 6 ("dimension size")) -> (w1987:u8[])
              n230 = Initialize Array(u8 32 ("y"), 6 ("dimension size")) -> (w1990:u8[])
              n231 = Initialize Array(u8 32 ("y"), 6 ("dimension size")) -> (w1989:u8[])
              n232 = local write "roll buffer"(w1987) -> ()
              n233 = local write "pitch buffer"(w1990) -> ()
              n234 = local write "heading buffer"(w1989) -> ()
              n235 = Equal?(x=w1998, y=u8 10) -> (x = y?=w1996:bool)
              n236 = Select(t=T10."Read heading" ("Main states"), s=w1996, f=T10."Search for LF" ("Main states")) -> (s? t:f=w1995:T10)
            }
            frame #1 {
              n237 = local read "Compass read count"() -> (w2001:i32)
              n238 = flat-sequence {
                tunnel: [w2006] -> w2000
                tunnel: [w2004] -> w1999
                tunnel: w2000 -> [w2008]
                tunnel: w1999 -> [w2007]
                frame #0 {
                  n239 = call "Tick Count"() -> ("Tick Count(mSec)"=w2006:u16)
                  n240 = Subtract(x=w2006, y="Compass Tick Count(mSec)") -> (x-y=w2004:u16)
                }
                frame #1 {
                  n241 = local write "Compass Tick Count(mSec)"(w2008) -> ()
                  "Compass Period (ms)" <- w2007
                }
              }
              n242 = case shown="10" w2002 {
                tunnel: [w2012 T10."Read heading" ("Main states") T10."Read pitch" ("Main states")] -> w2003
                tunnel: w2002 -> [w2013 _ _]
                tunnel: w2001 -> [w2011 _ _]
                frame #0 {
                  n243 = Greater Or Equal?(x=w2011, y=6) -> (x >= y?=w2009:bool)
                  n244 = case shown="True" w2009 {
                    tunnel: w2013 -> [w2015 _]
                    tunnel: [T10."Read heading" ("Main states") T10."Read pitch" ("Main states")] -> w2012
                    frame #0 {
                      n245 = local read "Compass read count"() -> (w2017:i32)
                      n246 = local read "heading buffer"() -> (w2018:u8[])
                      n247 = Increment(x=w2017) -> (x+1=w2019:i32)
                      n248 = Replace Array Subset(array=w2018, new element=w2015, index=w2017) -> (w2016:u8[])
                      n249 = local write "Compass read count"(w2019) -> ()
                      n250 = local write "heading buffer"(w2016) -> ()
                    }
                    frame #1 {
                      n251 = local write "Compass read count"(0 ("Read count")) -> ()
                      n252 = local read "heading buffer"() -> (w2022:u8[])
                      n253 = local write "heading data"(w2022) -> ()
                    }
                  }
                }
                frame #1 {
                  w2030 = 0 ("Comma count")
                  # "LF read"
                  n254 = local write "Compass comma count"(w2030) -> ()
                  n255 = local write "Compass read count"(w2030) -> ()
                  n256 = Initialize Array(u8 32 ("y"), 6 ("dimension size")) -> (w2031:u8[])
                  n257 = Initialize Array(u8 32 ("y"), 6 ("dimension size")) -> (w2025:u8[])
                  n258 = Initialize Array(u8 32 ("y"), 6 ("dimension size")) -> (w2024:u8[])
                  n259 = local write "heading buffer"(w2031) -> ()
                  n260 = local write "pitch buffer"(w2025) -> ()
                  n261 = local write "roll buffer"(w2024) -> ()
                }
                frame #2 {
                  # "Assumes data string does not contain commas"
                  n262 = local write "Compass read count"(0 ("Comma count")) -> ()
                  n263 = local read "heading buffer"() -> (w2038:u8[])
                  n264 = local read "Compass Heartbeat"() -> (w2035:bool)
                  n265 = local write "heading data"(w2038) -> ()
                  n266 = Not(x=w2035) -> (.not. x?=w2034:bool)
                  n267 = local write "Compass Heartbeat"(w2034) -> ()
                }
              }
            }
            frame #2 {
              n268 = local read "Compass read count"() -> (w2039:i32)
              n269 = case shown="44" w2040 {
                tunnel: [w2045 T10."Read heading" ("Main states") T10."Read roll" ("Main states")] -> w2041
                tunnel: w2040 -> [w2046 _ _]
                tunnel: w2039 -> [w2044 _ _]
                frame #0 {
                  n270 = Greater Or Equal?(x=w2044, y=6) -> (x >= y?=w2042:bool)
                  n271 = case shown="True" w2042 {
                    tunnel: w2046 -> [w2048 _]
                    tunnel: [T10."Read pitch" ("Main states") T10."Read roll" ("Main states")] -> w2045
                    frame #0 {
                      n272 = local read "Compass read count"() -> (w2050:i32)
                      n273 = local read "pitch buffer"() -> (w2051:u8[])
                      n274 = Increment(x=w2050) -> (x+1=w2052:i32)
                      n275 = Replace Array Subset(array=w2051, new element=w2048, index=w2050) -> (w2049:u8[])
                      n276 = local write "Compass read count"(w2052) -> ()
                      n277 = local write "pitch buffer"(w2049) -> ()
                    }
                    frame #1 {
                      n278 = local write "Compass read count"(0 ("Read count")) -> ()
                      n279 = local read "pitch buffer"() -> (w2055:u8[])
                      n280 = local write "pitch data"(w2055) -> ()
                    }
                  }
                }
                frame #1 {
                  w2063 = 0 ("Comma count")
                  # "LF read"
                  n281 = local write "Compass comma count"(w2063) -> ()
                  n282 = local write "Compass read count"(w2063) -> ()
                  n283 = Initialize Array(u8 32 ("y"), 6 ("dimension size")) -> (w2064:u8[])
                  n284 = Initialize Array(u8 32 ("y"), 6 ("dimension size")) -> (w2058:u8[])
                  n285 = Initialize Array(u8 32 ("y"), 6 ("dimension size")) -> (w2057:u8[])
                  n286 = local write "heading buffer"(w2064) -> ()
                  n287 = local write "pitch buffer"(w2058) -> ()
                  n288 = local write "roll buffer"(w2057) -> ()
                }
                frame #2 {
                  # "Assumes data string does not contain commas"
                  n289 = local write "Compass read count"(0 ("Comma count")) -> ()
                  n290 = local read "pitch buffer"() -> (w2071:u8[])
                  n291 = local read "Compass Heartbeat"() -> (w2068:bool)
                  n292 = local write "pitch data"(w2071) -> ()
                  n293 = Not(x=w2068) -> (.not. x?=w2067:bool)
                  n294 = local write "Compass Heartbeat"(w2067) -> ()
                }
              }
            }
            frame #3 {
              n295 = local read "Compass read count"() -> (w2072:i32)
              n296 = case shown="0, Default" w2073 {
                tunnel: [w2080 T10."Read heading" ("Main states") T10."Search for LF" ("Main states")] -> w2074
                tunnel: w2073 -> [w2081 _ _]
                tunnel: w2072 -> [w2079 _ _]
                frame #0 {
                  n297 = Greater Or Equal?(x=w2079, y=6) -> (x >= y?=w2077:bool)
                  n298 = local read "Compass Heartbeat"() -> (w2076:bool)
                  n299 = case shown="False" w2077 {
                    tunnel: w2081 -> [w2083 _]
                    tunnel: [T10."Read roll" ("Main states") T10."Read pitch" ("Main states")] -> w2080
                    frame #0 {
                      n300 = local read "Compass read count"() -> (w2085:i32)
                      n301 = local read "roll buffer"() -> (w2086:u8[])
                      n302 = Increment(x=w2085) -> (x+1=w2087:i32)
                      n303 = Replace Array Subset(array=w2086, new element=w2083, index=w2085) -> (w2084:u8[])
                      n304 = local write "Compass read count"(w2087) -> ()
                      n305 = local write "roll buffer"(w2084) -> ()
                    }
                    frame #1 {
                      n306 = local write "Compass read count"(0 ("Read count")) -> ()
                      n307 = local read "heading buffer"() -> (w2090:u8[])
                      n308 = local write "heading data"(w2090) -> ()
                    }
                  }
                  n309 = Not(x=w2076) -> (.not. x?=w2075:bool)
                  n310 = local write "Compass Heartbeat"(w2075) -> ()
                }
                frame #1 {
                  w2098 = 0 ("Comma count")
                  # "LF read"
                  n311 = local write "Compass comma count"(w2098) -> ()
                  n312 = local write "Compass read count"(w2098) -> ()
                  n313 = Initialize Array(u8 32 ("y"), 6 ("dimension size")) -> (w2099:u8[])
                  n314 = Initialize Array(u8 32 ("y"), 6 ("dimension size")) -> (w2093:u8[])
                  n315 = Initialize Array(u8 32 ("y"), 6 ("dimension size")) -> (w2092:u8[])
                  n316 = local write "heading buffer"(w2099) -> ()
                  n317 = local write "pitch buffer"(w2093) -> ()
                  n318 = local write "roll buffer"(w2092) -> ()
                }
                frame #2 {
                  # "Assumes data string does not contain commas"
                  n319 = local read "roll buffer"() -> (w2104:u8[])
                  n320 = local write "Compass read count"(0 ("Comma count")) -> ()
                  n321 = local write "roll data"(w2104) -> ()
                }
              }
            }
          }
        }
        "Compass error out" <- w1912
      }
    }
  }
  n322 = while {
    shift-right: [w2116] -> _
    shift-left: _ -> [w2115]
    shift-right: [w2112] -> _
    shift-left: 0 -> [w2113]
    shift-right: [w2105] -> _
    shift-left: 0 -> [w2111]
    shift-right: [w2109] -> _
    shift-left: 0 -> [w2110]
    shift-right: [w2106] -> _
    shift-left: 0 -> [w2108]
    stop <- FALSE ("stop 2") stop-if-true
    # "Low Pulse Indicator"
    # "Low Pulse Counter"
    # "High Pulse Counter"
    # "High Pulse Indicator"
    n323 = xnode "FPGA I/O Node"() -> ("Mod2/DIO1"=w2116:bool)  [unwired: 1 in, 1 out]
    n324 = Select(t=5, s=w2116, f=0) -> (s? t:f=→"Waveform Chart (Turn)":i32)
    n325 = case shown="False" w2116 {
      selector: w2116 -> [w2128 w2142]
      tunnel: w2115 -> [w2130 w2144]
      tunnel: w2113 -> [_ w2140]
      tunnel: [0 w2139] -> w2112
      tunnel: [w2126 w2138] -> w2105
      tunnel: w2111 -> [w2126 w2137]
      tunnel: w2110 -> [w2124 _]
      tunnel: [w2123 0] -> w2109
      tunnel: w2108 -> [w2122 w2136]
      tunnel: [w2121 w2136] -> w2106
      frame #0 {
        n326 = Not(x=w2130) -> (.not. x?=w2129:bool)
        n327 = And(x=w2128, y=w2129) -> (x .and. y?=w2127:bool)
        n328 = case shown="False" w2127 {
          tunnel: w2124 -> [w2133 w2134]
          tunnel: [w2132 w2134] -> w2123
          tunnel: w2122 -> [w2131 _]
          tunnel: [w2131 w2134] -> w2121
          frame #0 {
            # "Count Low Pulse"
            n329 = Increment(x=w2133) -> (x+1=w2132:i32)
          }
          frame #1 {
            # "Stop Counting"
          }
        }
      }
      frame #1 {
        n330 = Not(x=w2142) -> (.not. x?=w2143:bool)
        n331 = And(x=w2143, y=w2144) -> (x .and. y?=w2141:bool)
        n332 = case shown="True" w2141 {
          tunnel: w2140 -> [w2147 w2148]
          tunnel: [w2146 w2148] -> w2139
          tunnel: [w2145 w2148] -> w2138
          tunnel: w2137 -> [w2145 _]
          frame #0 {
            # "Count High Pulse Length"
            n333 = Increment(x=w2147) -> (x+1=w2146:i32)
          }
          frame #1 {
            # "Stop Counting"
          }
        }
      }
    }
    "High Pulse Length (Turn)" <- w2105
    "Low Pulse Length (Turn)" <- w2106
    n334 = call "Wait10"("Count(mSec)"=u32 1) -> ()  [unwired: 1 out]
    n335 = Add(x=w2106, y=w2105) -> (x+y=→"Pulse Period (Turn)":i32)
  }
  n336 = while {
    shift-right: [w2179] -> _
    shift-left: _ -> [w2178]
    shift-right: [w2175] -> _
    shift-left: 0 -> [w2176]
    shift-right: [w2168] -> _
    shift-left: 0 -> [w2174]
    shift-right: [w2172] -> _
    shift-left: 0 -> [w2173]
    shift-right: [w2169] -> _
    shift-left: 0 -> [w2171]
    stop <- FALSE ("stop") stop-if-true
    # "Low Pulse Indicator"
    # "Low Pulse Counter"
    # "High Pulse Counter"
    # "High Pulse Indicator"
    n337 = xnode "FPGA I/O Node"() -> ("Mod2/DIO0"=w2179:bool)  [unwired: 1 in, 1 out]
    n338 = Select(t=5, s=w2179, f=0) -> (s? t:f=→"Waveform Chart (Throttle)":i32)
    n339 = case shown="True" w2179 {
      selector: w2179 -> [w2191 w2205]
      tunnel: w2178 -> [w2193 w2207]
      tunnel: w2176 -> [_ w2203]
      tunnel: [0 w2202] -> w2175
      tunnel: [w2189 w2201] -> w2168
      tunnel: w2174 -> [w2189 w2200]
      tunnel: w2173 -> [w2187 _]
      tunnel: [w2186 0] -> w2172
      tunnel: w2171 -> [w2185 w2199]
      tunnel: [w2184 w2199] -> w2169
      frame #0 {
        n340 = Not(x=w2193) -> (.not. x?=w2192:bool)
        n341 = And(x=w2191, y=w2192) -> (x .and. y?=w2190:bool)
        n342 = case shown="False" w2190 {
          tunnel: w2187 -> [w2196 w2197]
          tunnel: [w2195 w2197] -> w2186
          tunnel: w2185 -> [w2194 _]
          tunnel: [w2194 w2197] -> w2184
          frame #0 {
            # "Count Low Pulse"
            n343 = Increment(x=w2196) -> (x+1=w2195:i32)
          }
          frame #1 {
            # "Stop Counting"
          }
        }
      }
      frame #1 {
        n344 = Not(x=w2205) -> (.not. x?=w2206:bool)
        n345 = And(x=w2206, y=w2207) -> (x .and. y?=w2204:bool)
        n346 = case shown="False" w2204 {
          tunnel: w2203 -> [w2210 w2211]
          tunnel: [w2209 w2211] -> w2202
          tunnel: [w2208 w2211] -> w2201
          tunnel: w2200 -> [w2208 _]
          frame #0 {
            # "Count High Pulse Length"
            n347 = Increment(x=w2210) -> (x+1=w2209:i32)
          }
          frame #1 {
            # "Stop Counting"
          }
        }
      }
    }
    "High Pulse Length (Throttle)" <- w2168
    "Low Pulse Length (Throttle)" <- w2169
    n348 = call "Wait9"("Count(mSec)"=u32 1) -> ()  [unwired: 1 out]
    n349 = Add(x=w2169, y=w2168) -> (x+y=→"Pulse Period (Throttle)":i32)
  }
  n350 = while {
    stop <- FALSE stop-if-true
    n351 = local read "Debounce Timeout"() -> (w2231:i32)
    n352 = xnode "FPGA I/O Node"() -> ("Mod2/DIO19"=w2233:bool)  [unwired: 1 in, 1 out]
    n353 = case shown="True" w2233 {
      tunnel: w2231 -> [_ w2254]
      frame #0 {
      }
      frame #1 {
        n354 = while {
          tunnel: w2254 -> [w2260]
          tunnel: [w2256] -> w2253
          i -> [w2261]
          stop <- w2259 stop-if-true
          n355 = xnode "FPGA I/O Node"() -> ("Mod2/DIO19"=w2258:bool)  [unwired: 1 in, 1 out]
          n356 = Not(x=w2258) -> (.not. x?=w2257:bool)
          n357 = Greater?(x=w2261, y=w2260) -> (0:w2256:bool)
          n358 = call "Loop Timer6"("Count(mSec)"=u16 1) -> ()  [unwired: 1 out]
          n359 = Or(x=w2257, y=w2256) -> (x .or. y?=w2259:bool)
        }
        "Debounced Init Switch" <- w2253
      }
    }
  }
  n360 = while {
    stop <- FALSE stop-if-true
    n361 = xnode "FPGA I/O Node"() -> ("Mod2/DIO20"=w2282:bool)  [unwired: 1 in, 1 out]
    n362 = case shown="True" w2282 {
      tunnel: "Debounce Timeout" -> [_ w2304]
      frame #0 {
      }
      frame #1 {
        n363 = while {
          tunnel: w2304 -> [w2310]
          tunnel: [w2306] -> w2303
          i -> [w2311]
          stop <- w2309 stop-if-true
          n364 = xnode "FPGA I/O Node"() -> ("Mod2/DIO20"=w2308:bool)  [unwired: 1 in, 1 out]
          n365 = Not(x=w2308) -> (.not. x?=w2307:bool)
          n366 = Greater?(x=w2311, y=w2310) -> (0:w2306:bool)
          n367 = call "Loop Timer5"("Count(mSec)"=u16 1) -> ()  [unwired: 1 out]
          n368 = Or(x=w2307, y=w2306) -> (x .or. y?=w2309:bool)
        }
        "Debounced Safety Switch" <- w2303
      }
    }
  }
  n369 = while {
    stop <- FALSE stop-if-true
    n370 = local read "Debounce Timeout"() -> (w2331:i32)
    n371 = xnode "FPGA I/O Node"() -> ("Mod2/DIO21"=w2333:bool)  [unwired: 1 in, 1 out]
    n372 = case shown="True" w2333 {
      tunnel: w2331 -> [_ w2354]
      frame #0 {
      }
      frame #1 {
        n373 = while {
          tunnel: w2354 -> [w2360]
          tunnel: [w2356] -> w2353
          i -> [w2361]
          stop <- w2359 stop-if-true
          n374 = xnode "FPGA I/O Node"() -> ("Mod2/DIO21"=w2358:bool)  [unwired: 1 in, 1 out]
          n375 = Not(x=w2358) -> (.not. x?=w2357:bool)
          n376 = Greater?(x=w2361, y=w2360) -> (0:w2356:bool)
          n377 = call "Loop Timer7"("Count(mSec)"=u16 1) -> ()  [unwired: 1 out]
          n378 = Or(x=w2357, y=w2356) -> (x .or. y?=w2359:bool)
        }
        "Debounced Go Button" <- w2353
      }
    }
  }
  n379 = while {
    stop <- FALSE stop-if-true
    n380 = local read "Debounce Timeout"() -> (w2381:i32)
    n381 = xnode "FPGA I/O Node"() -> ("Mod2/DIO27"=w2383:bool)  [unwired: 1 in, 1 out]
    n382 = case shown="True" w2383 {
      tunnel: w2381 -> [_ w2404]
      frame #0 {
      }
      frame #1 {
        n383 = while {
          tunnel: w2404 -> [w2410]
          tunnel: [w2406] -> w2403
          i -> [w2411]
          stop <- w2409 stop-if-true
          n384 = xnode "FPGA I/O Node"() -> ("Mod2/DIO27"=w2408:bool)  [unwired: 1 in, 1 out]
          n385 = Not(x=w2408) -> (.not. x?=w2407:bool)
          n386 = Greater?(x=w2411, y=w2410) -> (0:w2406:bool)
          n387 = call "Loop Timer19"("Count(mSec)"=u16 1) -> ()  [unwired: 1 out]
          n388 = Or(x=w2407, y=w2406) -> (x .or. y?=w2409:bool)
        }
        "Debounced SW1" <- w2403
      }
    }
  }
  n389 = while {
    stop <- FALSE stop-if-true
    n390 = local read "Debounce Timeout"() -> (w2431:i32)
    n391 = xnode "FPGA I/O Node"() -> ("Mod2/DIO28"=w2433:bool)  [unwired: 1 in, 1 out]
    n392 = case shown="True" w2433 {
      tunnel: w2431 -> [_ w2454]
      frame #0 {
      }
      frame #1 {
        n393 = while {
          tunnel: w2454 -> [w2460]
          tunnel: [w2456] -> w2453
          i -> [w2461]
          stop <- w2459 stop-if-true
          n394 = xnode "FPGA I/O Node"() -> ("Mod2/DIO28"=w2458:bool)  [unwired: 1 in, 1 out]
          n395 = Not(x=w2458) -> (.not. x?=w2457:bool)
          n396 = Greater?(x=w2461, y=w2460) -> (0:w2456:bool)
          n397 = call "Loop Timer20"("Count(mSec)"=u16 1) -> ()  [unwired: 1 out]
          n398 = Or(x=w2457, y=w2456) -> (x .or. y?=w2459:bool)
        }
        "Debounced SW2" <- w2453
      }
    }
  }
  n399 = while {
    stop <- FALSE stop-if-true
    n400 = local read "Debounce Timeout"() -> (w2481:i32)
    n401 = xnode "FPGA I/O Node"() -> ("Mod2/DIO31"=w2483:bool)  [unwired: 1 in, 1 out]
    n402 = case shown="True" w2483 {
      tunnel: w2481 -> [_ w2504]
      frame #0 {
      }
      frame #1 {
        n403 = while {
          tunnel: w2504 -> [w2510]
          tunnel: [w2506] -> w2503
          i -> [w2511]
          stop <- w2509 stop-if-true
          n404 = xnode "FPGA I/O Node"() -> ("Mod2/DIO31"=w2508:bool)  [unwired: 1 in, 1 out]
          n405 = Not(x=w2508) -> (.not. x?=w2507:bool)
          n406 = Greater?(x=w2511, y=w2510) -> (0:w2506:bool)
          n407 = call "Loop Timer21"("Count(mSec)"=u16 1) -> ()  [unwired: 1 out]
          n408 = Or(x=w2507, y=w2506) -> (x .or. y?=w2509:bool)
        }
        "Debounced BTTN1" <- w2503
      }
    }
  }
  n409 = xnode "FPGA I/O Property Node"("Baud Rate"=nicrio_cRIO-9871_BaudRateEnum."4800 bps" ("Baud Rate 4"), "Data Bits"=nicrio_cRIO-9871_DataBitsEnum."8" ("Data Bits 4"), "Stop Bits"=nicrio_cRIO-9871_StopBitsEnum."1" ("Stop Bits 4"), "Parity"=nicrio_cRIO-9871_ParityEnum."None" ("Parity 4"), "Flow Control"=nicrio_cRIO-9871_FlowControlEnum."None" ("Flow Control 4")) -> ("error out"=w33:errorcluster)  [unwired: 2 in, 1 out]
  n410 = flat-sequence {
    tunnel: [w2532] -> w34
    tunnel: w33 -> [w2532]
    frame #0 {
      n411 = call "Wait5"("Count(mSec)"=u32 100) -> ()  [unwired: 1 out]
    }
  }
  n412 = while {
    tunnel: w34 -> [w2541]
    tunnel: u8[] [36, 74, 79, 70, 70, 10, 13] -> [w2540]
    tunnel: u8[] [36, 62] -> [w2536]
    tunnel: [w2533] -> w32
    stop <- w2534 stop-if-true
    n413 = flat-sequence {
      tunnel: w2541 -> [w2545]
      tunnel: w2540 -> [w2544]
      tunnel: [w2543] -> w2539
      tunnel: w2539 -> [w2591]
      tunnel: [w2591] -> w2538
      frame #0 {
        n414 = xnode "FPGA I/O Method Node"("error in"=w2545) -> ("error out"=w2546:errorcluster)  [unwired: 1 in, 1 out]
        n415 = for {
          tunnel: w2544 -> [w2550] mode=indexing
          tunnel: w2546 -> [w2548]
          tunnel: [w2547] -> w2543
          n416 = xnode "FPGA I/O Method Node"("error in"=w2548, "Data"=w2550, "Timeout (ms)"=1) -> ("error out"=w2547:errorcluster)  [unwired: 1 in, 2 out]
        }
      }
      frame #1 {
        n417 = call "Wait4"("Count(mSec)"=u32 100) -> ()  [unwired: 1 out]
      }
    }
    n418 = for {
      N: 2 -> [_]
      tunnel: [w2594] -> w2537 mode=indexing
      tunnel: w2538 -> [w2593]
      tunnel: [w2592] -> w2533
      n419 = xnode "FPGA I/O Method Node"("error in"=w2593, "Timeout (ms)"=1) -> ("error out"=w2592:errorcluster, "Data"=w2594:u8)  [unwired: 1 in, 2 out]
    }
    n420 = Equal?(x=w2536, y=w2537) -> (x = y?=w2535:bool[])
    n421 = And Array Elements(Boolean array=w2535) -> (logical AND=w2534:bool)
    "Output Halted" <- w2534
  }
  n422 = while {
    stop <- FALSE stop-if-true
    n423 = flat-sequence {
      frame #0 {
        n424 = call "Interrupt3"("Wait Until Cleared"=TRUE, "IRQ Number"=u8 10) -> ()  [unwired: 1 out]
      }
      frame #1 {
        n425 = xnode "FPGA I/O Node"("Mod2/DIO8"=TRUE ("Mod2/DIO9")) -> ()  [unwired: 1 in, 1 out]
      }
      frame #2 {
        n426 = call "Wait11"("Count(mSec)"="That Was Easy Duration") -> ()  [unwired: 1 out]
      }
      frame #3 {
        n427 = xnode "FPGA I/O Node"("Mod2/DIO8"=FALSE ("Mod2/DIO9")) -> ()  [unwired: 1 in, 1 out]
      }
    }
  }
  n428 = while "Read Encoders Loop" {
    shift-right: [w2693] -> _
    shift-left: _ -> [w2697]
    shift-right: [w2692] -> _
    shift-left: _ -> [w2707]
    shift-right: [w2709] -> _
    shift-left: _ -> [w2710]
    shift-right: [w2704] -> _
    shift-left: _ -> [w2706]
    shift-right: [w2699] -> _
    shift-left: _ -> [w2705]
    shift-right: [w2694] -> _
    shift-left: _ -> [w2702]
    shift-right: [w2695] -> _
    shift-left: _ -> [w2701]
    shift-right: [w2696] -> _
    shift-left: _ -> [w2698]
    shift-right: [w2678] -> _
    shift-left: _ -> [w2679]
    shift-right: [w2664] -> _
    shift-left: _ -> [w2677]
    shift-right: [w2675] -> _
    shift-left: _ -> [w2676]
    shift-right: [w2673] -> _
    shift-left: _ -> [w2674]
    shift-right: [w2671] -> _
    shift-left: _ -> [w2672]
    shift-right: [w2669] -> _
    shift-left: _ -> [w2670]
    shift-right: [w2666] -> _
    shift-left: _ -> [w2668]
    shift-right: [w2665] -> _
    shift-left: _ -> [w2667]
    stop <- FALSE stop-if-true
    # "A  -> Current Quadrature Encoder Channel A value\nA' -> Last value of Quadrature Encoder Channel A\nB  -> Current Quadrature Encoder Channel B value\nB' -> Last value of Quadrature Encoder Channel B"
    # ">>Acceleration (last)>>"
    # "Start Time"
    # "A'"
    # "B"
    # "A'"
    # "A"
    # "B'"
    # "B"
    # ">>ChB>>"
    # ">>ChA>>"
    # ">>    Velocity (last)    >>"
    # ">>   Position (last)   >>"
    # "Time Now"
    # ">>Time Elapsed>>"
    # "A  -> Current Quadrature Encoder Channel A value\nA' -> Last value of Quadrature Encoder Channel A\nB  -> Current Quadrature Encoder Channel B value\nB' -> Last value of Quadrature Encoder Channel B"
    # ">>Acceleration (last)>>"
    # "Start Time"
    # "A'"
    # "B"
    # "A'"
    # "A"
    # "B'"
    # "B"
    # ">>ChB>>"
    # ">>ChA>>"
    # ">>    Velocity (last)    >>"
    # ">>   Position (last)   >>"
    # "Time Now"
    # ">>Time Elapsed>>"
    n429 = call "Tick Count3"() -> ("Tick Count(uSec)"=w2700:u32)
    n430 = call "Tick Count4"() -> ("Tick Count(uSec)"=w2691:u32)
    n431 = xnode "FPGA I/O Node"() -> ("Mod2/DIO10"=w2693:bool, "Mod2/DIO9"=w2709:bool)  [unwired: 2 in, 2 out]
    n432 = xnode "FPGA I/O Node"() -> ("Mod2/DIO11"=w2678:bool, "Mod2/DIO12"=w2664:bool)  [unwired: 2 in, 2 out]
    n433 = Select(t=w2700, s=w2706, f=w2705) -> (s? t:f=w2699:u32)
    n434 = Select(t=w2691, s=w2674, f=w2672) -> (s? t:f=w2671:u32)
    n435 = xnode ("Saturation Subtract2")("x"=w2700, "y"=w2699) -> ("x-y"=w2703:u32)
    n436 = xnode ("Saturation Subtract2")("x"=w2691, "y"=w2671) -> ("x-y"=w2690:u32)
    n437 = Exclusive Or(1:w2710, 2:w2693) -> (0:w2711:bool)
    n438 = Exclusive Or(1:w2677, 2:w2678) -> (0:w2688:bool)
    n439 = Exclusive Or(1:w2697, 2:w2693) -> (0:w2712:bool)
    n440 = Exclusive Or(1:w2710, 2:w2709) -> (0:w2713:bool)
    n441 = Exclusive Or(1:w2679, 2:w2678) -> (0:w2687:bool)
    n442 = Exclusive Or(1:w2677, 2:w2664) -> (0:w2686:bool)
    n443 = Select(t=0 ("32 bit"), s="Position Reset", f=w2707) -> (s? t:f=w2717:i32)
    n444 = Select(t=0 ("32 bit"), s="Position Reset", f=w2676) -> (s? t:f=w2682:i32)
    n445 = Select(t=-1 ("32 bit"), s=w2711, f=1 ("32 bit")) -> (s? t:f=w2716:i32)
    n446 = Select(t=-1 ("32 bit"), s=w2688, f=1 ("32 bit")) -> (s? t:f=w2683:i32)
    n447 = Or(x=w2712, y=w2713) -> (x .or. y?=w2708:bool)
    n448 = Or(x=w2687, y=w2686) -> (x .or. y?=w2689:bool)
    n449 = Add(x=w2716, y=w2717) -> (x+y=w2719:i32)
    n450 = Add(x=w2683, y=w2682) -> (x+y=w2680:i32)
    n451 = Greater Or Equal?(x=w2703, y="Velocity Interval (uSec)") -> (x >= y?=w2704:bool)
    n452 = Greater Or Equal?(x=w2690, y="Velocity Interval (uSec)") -> (x >= y?=w2673:bool)
    n453 = Select(t=w2719, s=w2708, f=w2717) -> (s? t:f=w2692:i32)
    "Right Position (Counts)" <- w2692
    n454 = Select(t=w2680, s=w2689, f=w2682) -> (s? t:f=w2675:i32)
    "Left Position (Counts)" <- w2675
    n455 = case shown="True" w2704 {
      tunnel: w2692 -> [_ w2827]
      tunnel: w2702 -> [w2824 w2831]
      tunnel: [w2826 w2830] -> w2695
      tunnel: w2701 -> [w2826 w2829]
      tunnel: [w2825 w2828] -> w2696
      tunnel: w2698 -> [w2825 _]
      tunnel: [w2824 w2827] -> w2694
      frame #0 {
      }
      frame #1 {
        n456 = Subtract(x=w2827, y=w2831) -> (x-y=w2830:i32)
        n457 = Subtract(x=w2830, y=w2829) -> (x-y=w2828:i32)
      }
    }
    "Right Acceleration (Counts/Interval)" <- w2696
    "Right Velocity (Counts/Interval)" <- w2695
    n458 = case shown="True" w2673 {
      tunnel: w2675 -> [_ w2771]
      tunnel: w2670 -> [w2768 w2775]
      tunnel: [w2770 w2774] -> w2665
      tunnel: w2667 -> [w2770 w2773]
      tunnel: [w2769 w2772] -> w2666
      tunnel: w2668 -> [w2769 _]
      tunnel: [w2768 w2771] -> w2669
      frame #0 {
      }
      frame #1 {
        n459 = Subtract(x=w2771, y=w2775) -> (x-y=w2774:i32)
        n460 = Subtract(x=w2774, y=w2773) -> (x-y=w2772:i32)
      }
    }
    "Left Acceleration (Counts/Interval)" <- w2666
    "Left Velocity (Counts/Interval)" <- w2665
  }
  n461 = while {
    tunnel: w32 -> [w2840]
    tunnel: u8[] [36, 74, 65, 83, 67, 44, 71, 80, 71, 71, 65, 44, 49, 48, 10, 13] -> [w2839]
    tunnel: u8[] [36, 62] -> [w2835]
    tunnel: [w2832] -> w29
    stop <- w2833 stop-if-true
    n462 = flat-sequence {
      tunnel: w2840 -> [w2842]
      tunnel: w2839 -> [w2844]
      tunnel: [w2843] -> w2838
      tunnel: w2838 -> [w2890]
      tunnel: [w2890] -> w2837
      frame #0 {
        n463 = xnode "FPGA I/O Method Node"("error in"=w2842) -> ("error out"=w2845:errorcluster)  [unwired: 1 in, 1 out]
        n464 = for {
          tunnel: w2844 -> [w2849] mode=indexing
          tunnel: w2845 -> [w2847]
          tunnel: [w2846] -> w2843
          n465 = xnode "FPGA I/O Method Node"("error in"=w2847, "Data"=w2849, "Timeout (ms)"=1) -> ("error out"=w2846:errorcluster)  [unwired: 1 in, 2 out]
        }
      }
      frame #1 {
        n466 = call "Wait6"("Count(mSec)"=u32 100) -> ()  [unwired: 1 out]
      }
    }
    n467 = for {
      N: 2 -> [_]
      tunnel: [w2893] -> w2836 mode=indexing
      tunnel: w2837 -> [w2892]
      tunnel: [w2891] -> w2832
      n468 = xnode "FPGA I/O Method Node"("error in"=w2892, "Timeout (ms)"=1) -> ("error out"=w2891:errorcluster, "Data"=w2893:u8)  [unwired: 1 in, 2 out]
    }
    n469 = Equal?(x=w2835, y=w2836) -> (x = y?=w2834:bool[])
    n470 = And Array Elements(Boolean array=w2834) -> (logical AND=w2833:bool)
    "Output Started" <- w2833
  }
  n471 = while {
    tunnel: w29 -> [w2943]
    shift-right: [w2934] -> _
    shift-left: u8[] [0, 0, 0, 0, 0, 0] -> [w2937]
    tunnel: u8[] [36, 71, 80, 71, 71, 65] -> [w2936]
    stop <- FALSE stop-if-true
    n472 = while {
      tunnel: w2943 -> [w3071]
      tunnel: [w3070] -> w2942
      tunnel: [w3069] -> w2935
      i -> [w3076]
      stop <- w3075 stop-if-true
      n473 = xnode "FPGA I/O Property Node"("error in"=w3071) -> ("error out"=w3070:errorcluster, "Bytes at Port"=w3073:u8)  [unwired: 1 in, 1 out]
      n474 = call "Loop Timer8"("Count(uSec)"=u32 1) -> ()  [unwired: 1 out]
      n475 = Greater Than 0?(x=w3073) -> (x > 0?=w3069:bool)
      "Bytes at Port?" <- w3069
      n476 = Greater Or Equal?(x=w3076, y="GPS Read Timeout (us)") -> (x >= y?=w3074:bool)
      n477 = Or(x=w3074, y=w3069) -> (x .or. y?=w3075:bool)
    }
    n478 = case shown="True" w2935 {
      tunnel: w2942 -> [w2945 w2954]
      tunnel: [w2945 w2952] -> w2940
      tunnel: w2937 -> [w2944 w2948]
      tunnel: [w2944 w2949] -> w2933
      frame #0 {
      }
      frame #1 {
        n479 = xnode "FPGA I/O Method Node"("error in"=w2954, "Timeout (ms)"=1) -> ("error out"=w2952:errorcluster, "Data"=w2951:u8)  [unwired: 1 in, 2 out]
        n480 = Rotate 1D Array(1:w2948, 2:5 ("n")) -> (0:w2947:u8[])
        n481 = Replace Array Subset(array=w2947, new element=w2951, index=5) -> (w2949:u8[])
      }
    }
    n482 = Equal?(x=w2936, y=w2933) -> (x = y?=w2941:bool[])
    n483 = And Array Elements(Boolean array=w2941) -> (logical AND=w2939:bool)
    "New GPS Data" <- w2939
    n484 = case shown="False" w2939 {
      tunnel: w2940 -> [w2992 w2997]
      tunnel: [w2993 u8[] [0, 0, 0, 0, 0, 0]] -> w2934
      tunnel: w2933 -> [w2993 _]
      tunnel: [w2992 w2994] -> w2932
      frame #0 {
      }
      frame #1 {
        n485 = for {
          N: 50 -> [_]
          tunnel: w2997 -> [w3003]
          tunnel: [w3000] -> w2996 mode=indexing
          tunnel: [w2999] -> w2994
          n486 = while {
            tunnel: w3003 -> [w3007]
            tunnel: [w3006] -> w3002
            i -> [w3011]
            stop <- w3010 stop-if-true
            n487 = local read "GPS Read Timeout (us)"() -> (w3004:i32)
            n488 = xnode "FPGA I/O Property Node"("error in"=w3007) -> ("error out"=w3006:errorcluster, "Bytes at Port"=w3008:u8)  [unwired: 1 in, 1 out]
            n489 = call "Loop Timer9"("Count(uSec)"=u32 1) -> ()  [unwired: 1 out]
            n490 = Greater Than 0?(x=w3008) -> (x > 0?=w3005:bool)
            n491 = Greater Or Equal?(x=w3011, y=w3004) -> (x >= y?=w3009:bool)
            n492 = Or(x=w3009, y=w3005) -> (x .or. y?=w3010:bool)
          }
          n493 = xnode "FPGA I/O Method Node"("error in"=w3002, "Timeout (ms)"=1) -> ("error out"=w2999:errorcluster, "Data"=w3000:u8)  [unwired: 1 in, 2 out]
        }
        "GPS Data" <- w2996
      }
    }
    "GPS error out" <- w2932
    "Current Buffer" <- w2937
  }
